vi "GetVoltage.vi"(4 "error in":errorcluster, 5 "connection ID":refnum<k5>) -> (0 "Voltage":string, 1 "error out":errorcluster, 2 "connection ID out":refnum<k5>, 3 "Answer":bool)   [LabVIEW 2013]
panel:
  out "читаю hex":string
  out "читаю текст":string
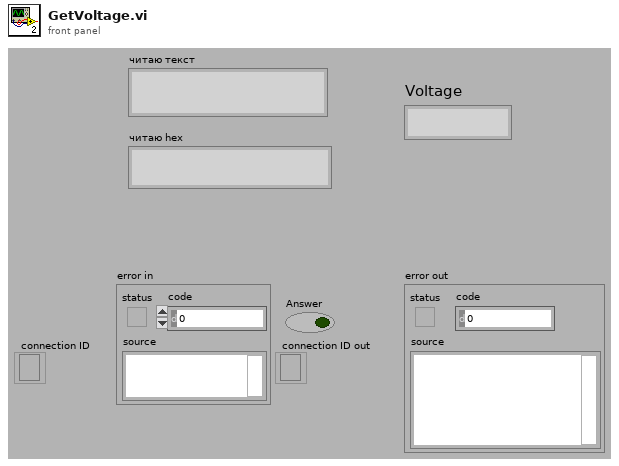
[diagram p1: front panel]
types:
  T1 = enum16{"Standard", "Buffered", "CRLF", "Immediate"}
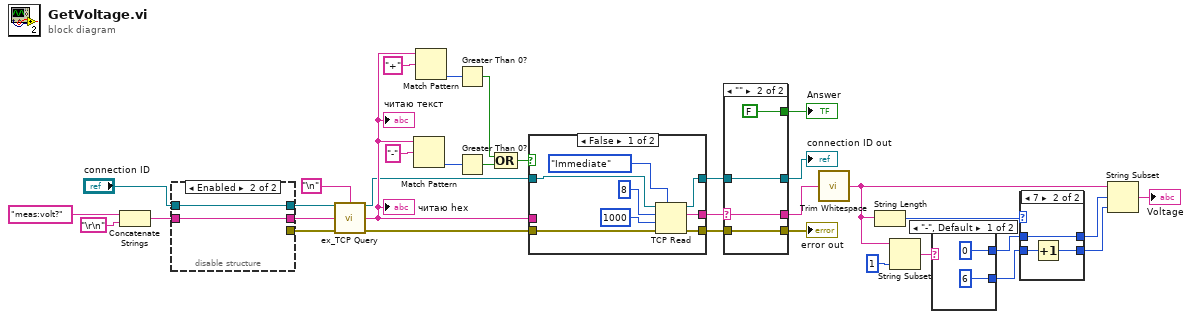
[diagram p0: block diagram]
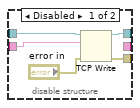
[diagram p2: hidden frame]
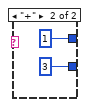
[diagram p4: hidden frame]
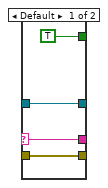
[diagram p6: hidden frame]
diagram:
  n1 = Concatenate Strings("meas:volt?" ("data in"), "\r\n") -> (w32:string)
  n2 = disable-structure shown="Enabled" {
    disable-tunnel: "connection ID" -> [w38 w40]
    disable-tunnel: w32 -> [w37 w41]
    disable-tunnel: [w36 _] -> w7
    disable-tunnel: [w35 w40] -> w6
    disable-tunnel: [_ w41] -> w5
    frame Disabled {
      n3 = TCP Write(connection ID=w38, data in=w37, error in (no error)="error in") -> (connection ID out=w35:refnum<k5>, error out=w36:errorcluster)  [unwired: 2 out]
    }
    frame Enabled {
    }
  }
  n4 = call "ex_TCP Query.vi"("TCP Network Connection in"=w6, "Termination character"="\n", "Query string"=w5, "error in (no error)"=w7) -> ("TCP Network Connection out"=w2:refnum<k5>, "Message data out"=w3:string, "error out"=w4:errorcluster)  [unwired: 8 in, 1 out]
  "читаю hex" <- w3
  "читаю текст" <- w3
  n5 = Match Pattern(string=w3, regular expression="-") -> (offset past match=w21:i32)  [unwired: 1 in, 3 out]
  n6 = Match Pattern(string=w3, regular expression="+") -> (offset past match=w29:i32)  [unwired: 1 in, 3 out]
  n7 = Greater Than 0?(x=w29) -> (x > 0?=w20:bool)
  n8 = Greater Than 0?(x=w21) -> (x > 0?=w19:bool)
  n9 = Compound Arithmetic op=OR(w20, w19) -> (w18:bool)
  n10 = case shown="False" w18 {
    tunnel: w3 -> [_ w52]
    tunnel: [w46 w52] -> w25
    tunnel: [w44 w50] -> w24
    tunnel: w4 -> [w45 w50]
    tunnel: w2 -> [w47 w51]
    tunnel: [w42 w51] -> w23
    frame False {
      n11 = TCP Read(connection ID=w47, bytes to read=8, error in (no error)=w45, 7:T1."Immediate" ("mode (standard)"), 9:1000 ("timeout ms (25000)")) -> (connection ID out=w42:refnum<k5>, data out=w46:string, error out=w44:errorcluster)
    }
    frame True {
    }
  }
  n12 = case shown="\"\"" w25 {
    selector: w25 -> [w56 w60]
    tunnel: [w56 w60] -> w8
    tunnel: [TRUE FALSE] -> w26
    tunnel: w24 -> [w54 w58]
    tunnel: [w54 w58] -> w27
    tunnel: w23 -> [w53 w57]
    tunnel: [w53 w57] -> w28
    frame Default {
    }
    frame "" {
    }
  }
  "Answer" <- w26
  "connection ID out" <- w28
  "error out" <- w27
  n13 = call <vilib>:"Trim Whitespace.vi"("string"=w8) -> ("trimmed string"=w15:string)  [unwired: 1 in]
  n14 = String Length(string=w15) -> (length=w14:i32)
  n15 = String Subset(string=w15, length (rest)=1 ("length (rest)")) -> (substring=w17:string)  [unwired: 1 in]
  n16 = case shown="\"-\", Default" w17 {
    tunnel: [0 ("length (rest)") 1 ("length (rest)")] -> w11
    tunnel: [6 ("length (rest)") 3 ("length (rest)")] -> w13
    frame "-", Default {
    }
    frame "+" {
    }
  }
  n17 = case shown="7" w14 {
    tunnel: w13 -> [w66 w69]
    tunnel: [w66 w68] -> w12
    tunnel: w11 -> [w65 w67]
    tunnel: [w65 w67] -> w10
    frame 6, Default {
    }
    frame 7 {
      n18 = Increment(x=w69) -> (x+1=w68:i32)
    }
  }
  n19 = String Subset(string=w15, offset (0)=w10, length (rest)=w12) -> (substring=→"Voltage":string)
